vi "degrees_to_radians.vi"(1 "degrees":dbl format="%.2f") -> (0 "radians":dbl format="%.2f")   [LabVIEW 2010]
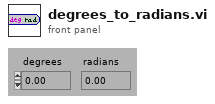
[diagram p1: front panel]
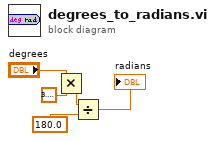
[diagram p0: block diagram]
diagram:
  n1 = Multiply(x="degrees", y=3.141592653589793) -> (x*y=w5:dbl)
  n2 = Divide(x=w5, y=180.0) -> (x/y=→"radians":dbl)
